vi "Display Discrete Probability Distributions.vi"() -> ()   [LabVIEW 2023]
doc: "This example VI uses Discrete PF , Discrete CDF , Discrete Inverse CDF VIs to display discrete probability (mass) functions, cumulative distribution functions, and inverse cumulative distribution functions for several discrete distributions."
uses:
  <vilib>/gmath/statdist.llb/Binomial Moments.vi
  <vilib>/gmath/statdist.llb/Binomial PF.vi
  <vilib>/gmath/statdist.llb/Binomial CDF.vi
  <vilib>/gmath/statdist.llb/Binomial Inverse CDF.vi
  <vilib>/gmath/statdist.llb/Bernoulli Moments.vi
  <vilib>/gmath/statdist.llb/Bernoulli CDF.vi
  <vilib>/gmath/statdist.llb/Bernoulli Inverse CDF.vi
  <vilib>/gmath/statdist.llb/Bernoulli PF.vi
  <vilib>/gmath/statdist.llb/Geometric Moments.vi
  <vilib>/gmath/statdist.llb/Geometric PF.vi
  <vilib>/gmath/statdist.llb/Geometric CDF.vi
  <vilib>/gmath/statdist.llb/Geometric Inverse CDF.vi
  <vilib>/gmath/statdist.llb/Hypergeometric Moments.vi
  <vilib>/gmath/statdist.llb/Hypergeometric PF.vi
  <vilib>/gmath/statdist.llb/Hypergeometric CDF.vi
  <vilib>/gmath/statdist.llb/Hypergeometric Inverse CDF.vi
  <vilib>/gmath/statdist.llb/Neg Binomial Moments.vi
  <vilib>/gmath/statdist.llb/Neg Binomial CDF.vi
  <vilib>/gmath/statdist.llb/Neg Binomial Inverse CDF.vi
  <vilib>/gmath/statdist.llb/Neg Binomial PF.vi
  <vilib>/gmath/statdist.llb/Poisson Moments.vi
  <vilib>/gmath/statdist.llb/Poisson PF.vi
  <vilib>/gmath/statdist.llb/Poisson CDF.vi
  <vilib>/gmath/statdist.llb/Poisson Inverse CDF.vi
  <vilib>/gmath/NI_Gmath.lvlib
panel:
  in  "Stop":bool
  in  "Tab Control":T1(tab)
  out "Bernoulli Inverse Cumulative Distribution Function":cluster{dbl[], i32[]}(graph)
  out "Bernoulli Cumulative Distribution Function":cluster{i32[], dbl[]}(graph)
  out "Variance (Bernoulli)":dbl
  out "Mean (Bernoulli)":dbl
  out "Bernoulli Probability Function":cluster{i32[], dbl[]}(graph)
  in  "p (Bernoulli)":dbl(slide)=0.3 min=0.0 max=1.0 scale=0.0..1.0
  out "Variance (Binomial)":dbl
  out "Mean (Binomial)":dbl
  in  "end (Binomial)":i32=20
  in  "start (Binomial)":i32
  in  "n (Binomial)":i32=13
  in  "p (Binomial)":dbl(slide)=0.3 min=0.0 max=1.0 scale=0.0..1.0
  out "Binomial Cumulative Distribution Function":cluster{i32[], dbl[]}(graph)
  out "Binomial Inverse Cumulative Distribution Function":cluster{dbl[], i32[]}(graph)
  out "Binomial Probability Function":cluster{i32[], dbl[]}(graph)
  in  "start (Geometric)":i32
  in  "end (Geometric)":i32=35
  out "Geometric Inverse Cumulative Distribution Function":cluster{dbl[], i32[]}(graph)
  out "Geometric Cumulative Distribution Function":cluster{i32[], dbl[]}(graph)
  out "Variance (Geometric)":dbl
  out "Mean (Geometric)":dbl
  out "Geometric Probability Function":cluster{i32[], dbl[]}(graph)
  in  "p (Geometric)":dbl(slide)=0.2 min=0.0 max=1.0 scale=0.0..1.0
  out "Variance (Hyper)":dbl
  out "Mean (Hyper)":dbl
  in  "n (Hyper)":i32=20
  in  "start (Hyper)":i32
  in  "end (Hyper)":i32=20
  in  "M (Hyper)":i32=31
  in  "k (Hyper)":i32=14
  out "Hypergeometric Cumulative Distribution Function":cluster{i32[], dbl[]}(graph)
  out "Hypergeometric Inverse Cumulative Distribution Function":cluster{dbl[], i32[]}(graph)
  out "Hypergeometric Probability Function":cluster{i32[], dbl[]}(graph)
  in  "start (Neg Binomial)":i32
  in  "end (Neg Binomial)":i32=40
  out "Neg Binomial Inverse Cumulative Distribution Function":cluster{dbl[], i32[]}(graph)
  in  "n (Neg Binomial)":i32=7
  out "Neg Binomial Cumulative Distribution Function":cluster{i32[], dbl[]}(graph)
  out "Variance (Neg Binomial)":dbl
  out "Mean (Neg Binomial)":dbl
  out "Neg Binomial Probability Function":cluster{i32[], dbl[]}(graph)
  in  "p (Neg Binomial)":dbl(slide)=0.4 min=0.0 max=1.0 scale=0.0..1.0
  out "Variance (Poisson)":dbl
  out "Mean (Poisson)":dbl
  in  "Lambda (Poisson)":dbl(slide)=22.0 scale=1e-08..50.0
  in  "end (Poisson)":i32=50
  in  "start (Poisson)":i32
  out "Poisson Inverse Cumulative Distribution Function":cluster{dbl[], i32[]}(graph)
  out "Poisson Cumulative Distribution Function":cluster{i32[], dbl[]}(graph)
  out "Poisson Probability Function":cluster{i32[], dbl[]}(graph)
  # "Overview: Demonstrates the use of the Discrete PF VI, Discrete CDF VI, and Discrete Inverse CDF VI.\nRequirements: LabVIEW Full Development System\nInstructions: \n1. Run the VI.\n2. Switch between tabs to explore how the parameters affect each distribution.\n3. Click Stop to stop the VI."
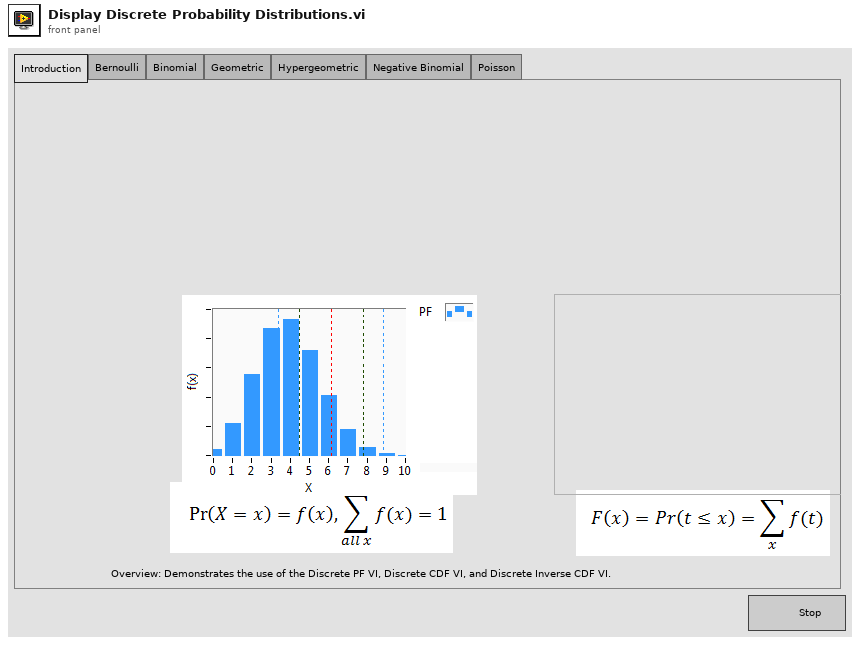
[diagram p1: front panel]
types:
  T1 = enum32{"Introduction", "Bernoulli", "Binomial", "Geometric", "Hypergeometric", "Negative Binomial", "Poisson"}
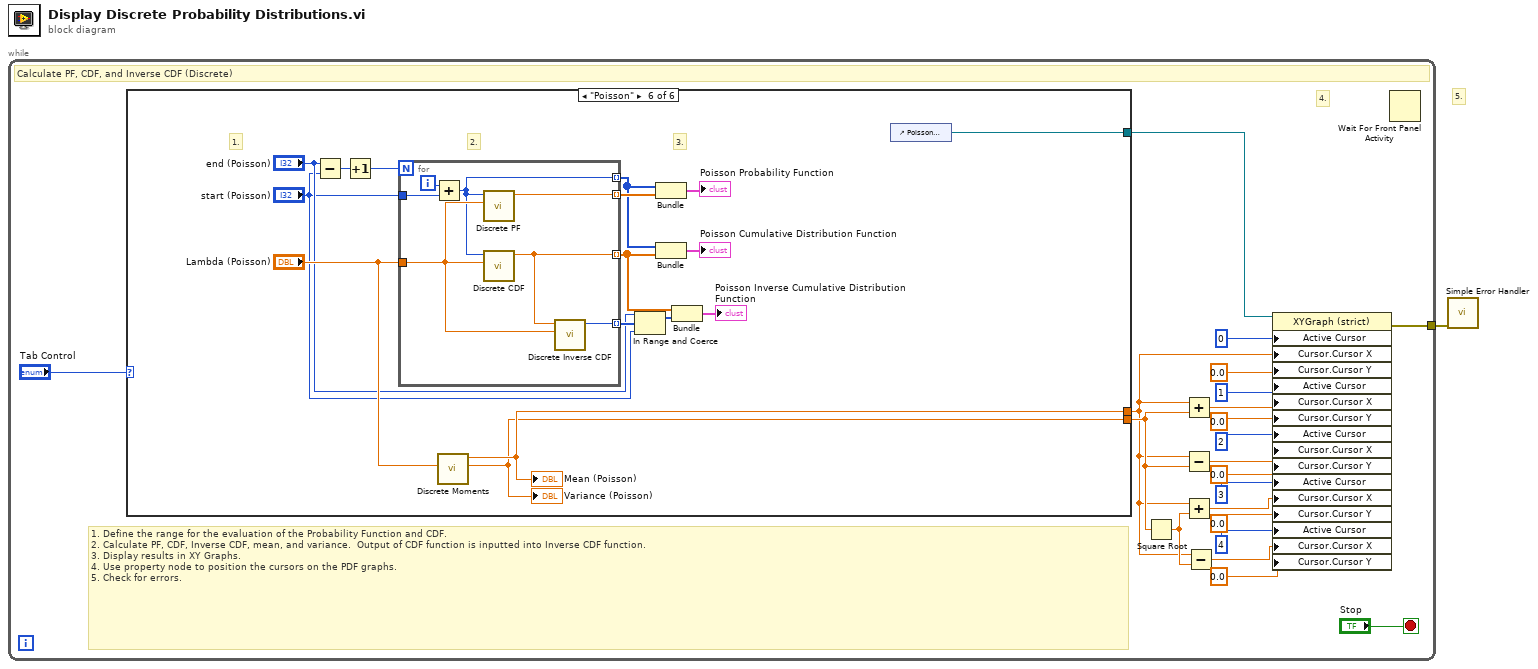
[diagram p0: block diagram]
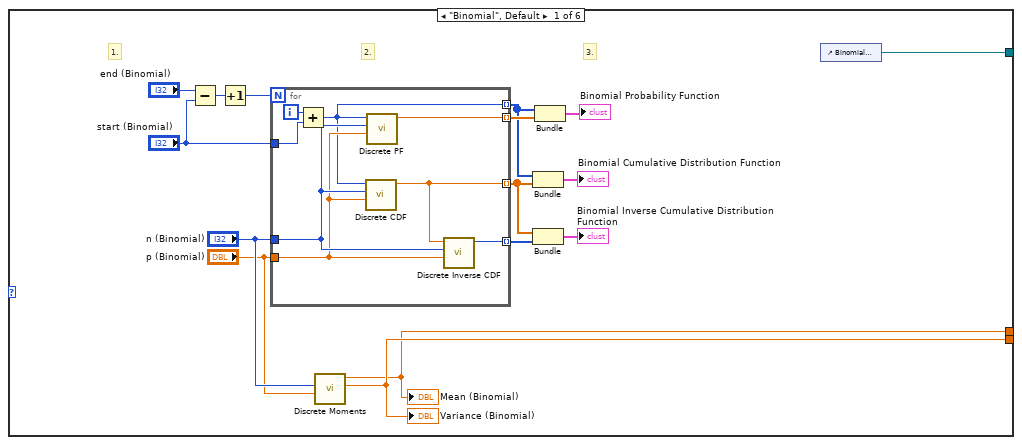
[diagram p2: hidden frame]
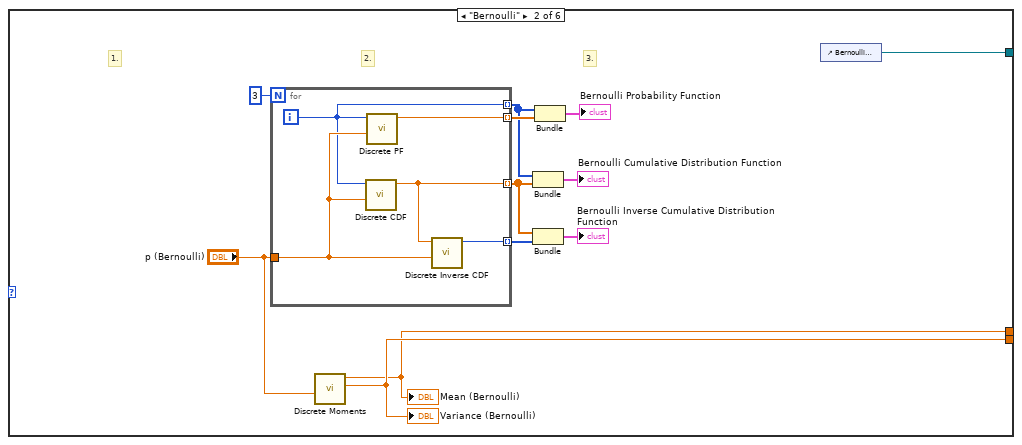
[diagram p3: hidden frame]
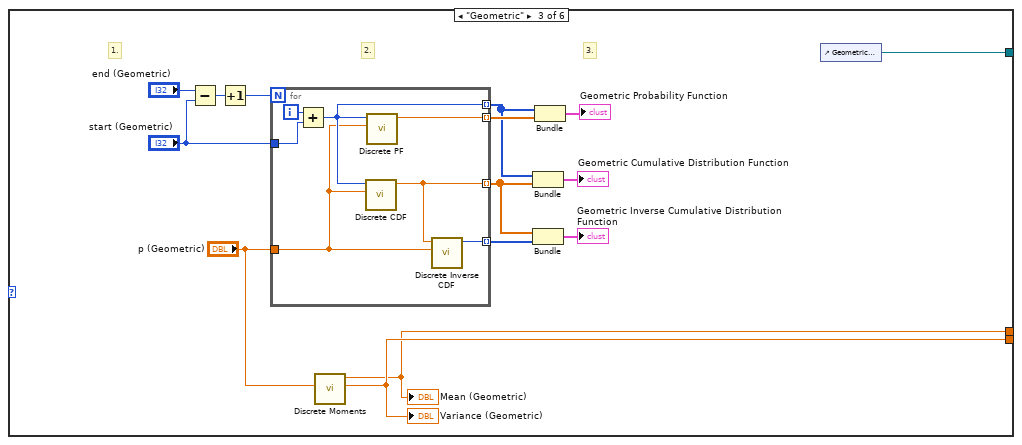
[diagram p4: hidden frame]
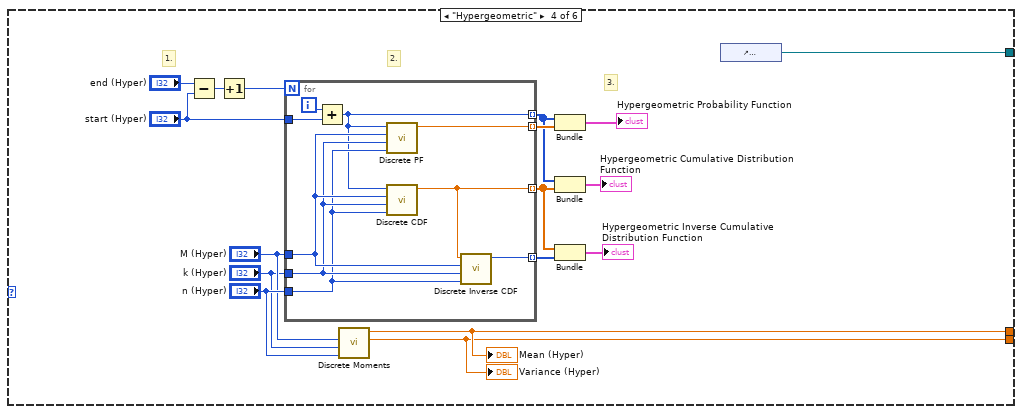
[diagram p5: hidden frame]
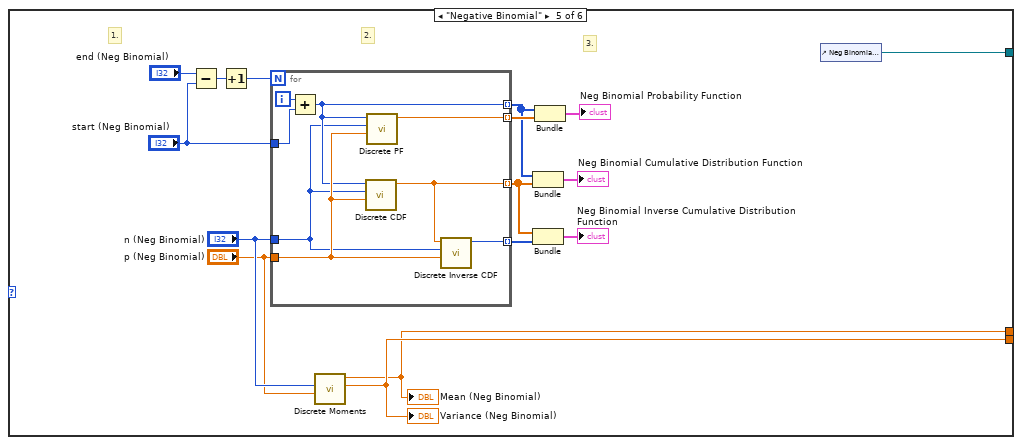
[diagram p6: hidden frame]
diagram:
  # "5."
  n1 = while {
    tunnel: [w4] -> w1
    stop <- "Stop" stop-if-true
    # "1. Define the range for the evaluation of the Probability Function and CDF.\n2. Calculate PF, CDF, Inverse CDF, mean, and variance.  Output of CDF function is inputted into Inverse CDF function.\n3. Display results in XY Graphs.\n4. Use property node to position the cursors on the PDF graphs.\n5. Check for errors."
    # "4."
    # "Calculate PF, CDF, and Inverse CDF (Discrete)"
    n2 = case shown="\"Poisson\"" "Tab Control" {
      tunnel: [w28 w49 w70 w95 w117 w144] -> w2
      tunnel: [w29 w50 w71 w94 w118 w143] -> w5
      tunnel: [w30 w51 w72 w93 w119 w145] -> w3
      frame "Binomial", Default {
        # "3."
        # "2."
        # "1."
        n3 = Subtract(x="end (Binomial)", y="start (Binomial)") -> (x-y=w24:i32)
        n4 = Increment(x=w24) -> (x+1=w23:i32)
        n5 = for {
          N: w23 -> [_]
          tunnel: [w46] -> w38 mode=indexing
          tunnel: [w44] -> w36 mode=indexing
          tunnel: [w45] -> w37 mode=indexing
          tunnel: "n (Binomial)" -> [w43]
          tunnel: "p (Binomial)" -> [w42]
          tunnel: "start (Binomial)" -> [w40]
          tunnel: [w39] -> w27 mode=indexing
          i -> [w41]
          n6 = Add(x=w41, y=w40) -> (x+y=w39:i32)
          n7 = call-poly <vilib>:"Discrete CDF.vi"("p"=w42, "n"=w43, "x"=w39) -> ("cdf(x)"=w44:dbl)  [unwired: 7 in, 1 out]
          n8 = call-poly <vilib>:"Discrete PF.vi"("p"=w42, "n"=w43, "x"=w39) -> ("prob(x)"=w46:dbl)  [unwired: 7 in, 1 out]
          n9 = call-poly <vilib>:"Discrete Inverse CDF.vi"("p"=w42, "n"=w43, "cdf(x)"=w44) -> ("x"=w45:i32)  [unwired: 7 in, 1 out]
        }
        n10 = call-poly <vilib>:"Discrete Moments.vi"("p"="p (Binomial)", "n"="n (Binomial)") -> ("variance"=w29:dbl, "mean"=w28:dbl)  [unwired: 7 in, 1 out]
        "Mean (Binomial)" <- w28
        "Variance (Binomial)" <- w29
        n11 = Bundle(w27, w36) -> (→"Binomial Cumulative Distribution Function":cluster{i32[], dbl[]})  [unwired: 1 in]
        n12 = Bundle(w36, w37) -> (→"Binomial Inverse Cumulative Distribution Function":cluster{dbl[], i32[]})  [unwired: 1 in]
        n13 = Bundle(w27, w38) -> (→"Binomial Probability Function":cluster{i32[], dbl[]})  [unwired: 1 in]
        n14 = control-ref of="Binomial Probability Function"() -> (w30:refnum<vi>)
      }
      frame "Bernoulli" {
        # "3."
        # "2."
        # "1."
        n15 = for {
          N: 3 -> [_]
          tunnel: [w63] -> w58 mode=indexing
          tunnel: [w61] -> w56 mode=indexing
          tunnel: [w62] -> w57 mode=indexing
          tunnel: "p (Bernoulli)" -> [w60]
          tunnel: [w59] -> w48 mode=indexing
          i -> [w59]
          n16 = call-poly <vilib>:"Discrete CDF.vi"("p"=w60, "x"=w59) -> ("cdf(x)"=w61:dbl)  [unwired: 8 in, 1 out]
          n17 = call-poly <vilib>:"Discrete PF.vi"("p"=w60, "x"=w59) -> ("prob(x)"=w63:dbl)  [unwired: 8 in, 1 out]
          n18 = call-poly <vilib>:"Discrete Inverse CDF.vi"("p"=w60, "cdf(x)"=w61) -> ("x"=w62:i32)  [unwired: 8 in, 1 out]
        }
        n19 = call-poly <vilib>:"Discrete Moments.vi"("p"="p (Bernoulli)") -> ("variance"=w50:dbl, "mean"=w49:dbl)  [unwired: 8 in, 1 out]
        "Mean (Bernoulli)" <- w49
        "Variance (Bernoulli)" <- w50
        n20 = Bundle(w48, w56) -> (→"Bernoulli Cumulative Distribution Function":cluster{i32[], dbl[]})  [unwired: 1 in]
        n21 = Bundle(w56, w57) -> (→"Bernoulli Inverse Cumulative Distribution Function":cluster{dbl[], i32[]})  [unwired: 1 in]
        n22 = Bundle(w48, w58) -> (→"Bernoulli Probability Function":cluster{i32[], dbl[]})  [unwired: 1 in]
        n23 = control-ref of="Bernoulli Probability Function"() -> (w51:refnum<vi>)
      }
      frame "Geometric" {
        # "3."
        # "2."
        # "1."
        n24 = Subtract(x="end (Geometric)", y="start (Geometric)") -> (x-y=w66:i32)
        n25 = Increment(x=w66) -> (x+1=w65:i32)
        n26 = for {
          N: w65 -> [_]
          tunnel: [w85] -> w78 mode=indexing
          tunnel: [w83] -> w76 mode=indexing
          tunnel: [w84] -> w77 mode=indexing
          tunnel: "p (Geometric)" -> [w79]
          tunnel: "start (Geometric)" -> [w81]
          tunnel: [w80] -> w69 mode=indexing
          i -> [w82]
          n27 = Add(x=w82, y=w81) -> (x+y=w80:i32)
          n28 = call-poly <vilib>:"Discrete CDF.vi"("p"=w79, "n"=w80) -> ("cdf(n)"=w83:dbl)  [unwired: 8 in, 1 out]
          n29 = call-poly <vilib>:"Discrete PF.vi"("p"=w79, "x"=w80) -> ("prob(x)"=w85:dbl)  [unwired: 8 in, 1 out]
          n30 = call-poly <vilib>:"Discrete Inverse CDF.vi"("p"=w79, "cdf(n)"=w83) -> ("n"=w84:i32)  [unwired: 8 in, 1 out]
        }
        n31 = call-poly <vilib>:"Discrete Moments.vi"("p"="p (Geometric)") -> ("variance"=w71:dbl, "mean"=w70:dbl)  [unwired: 8 in, 1 out]
        "Mean (Geometric)" <- w70
        "Variance (Geometric)" <- w71
        n32 = Bundle(w69, w76) -> (→"Geometric Cumulative Distribution Function":cluster{i32[], dbl[]})  [unwired: 1 in]
        n33 = Bundle(w76, w77) -> (→"Geometric Inverse Cumulative Distribution Function":cluster{dbl[], i32[]})  [unwired: 1 in]
        n34 = Bundle(w69, w78) -> (→"Geometric Probability Function":cluster{i32[], dbl[]})  [unwired: 1 in]
        n35 = control-ref of="Geometric Probability Function"() -> (w72:refnum<vi>)
      }
      frame "Hypergeometric" {
        # "3."
        # "2."
        # "1."
        n36 = Subtract(x="end (Hyper)", y="start (Hyper)") -> (x-y=w90:i32)
        n37 = Increment(x=w90) -> (x+1=w88:i32)
        n38 = for {
          N: w88 -> [_]
          tunnel: [w111] -> w102 mode=indexing
          tunnel: [w109] -> w100 mode=indexing
          tunnel: [w110] -> w101 mode=indexing
          tunnel: "M (Hyper)" -> [w108]
          tunnel: "k (Hyper)" -> [w107]
          tunnel: "n (Hyper)" -> [w106]
          tunnel: "start (Hyper)" -> [w104]
          tunnel: [w103] -> w86 mode=indexing
          i -> [w105]
          n39 = Add(x=w105, y=w104) -> (x+y=w103:i32)
          n40 = call-poly <vilib>:"Discrete PF.vi"("n"=w106, "k"=w107, "M"=w108, "x"=w103) -> ("prob(x)"=w111:dbl)  [unwired: 6 in, 1 out]
          n41 = call-poly <vilib>:"Discrete CDF.vi"("n"=w106, "k"=w107, "M"=w108, "x"=w103) -> ("cdf(x)"=w109:dbl)  [unwired: 6 in, 1 out]
          n42 = call-poly <vilib>:"Discrete Inverse CDF.vi"("n"=w106, "k"=w107, "M"=w108, "cdf(x)"=w109) -> ("x"=w110:i32)  [unwired: 6 in, 1 out]
        }
        n43 = call-poly <vilib>:"Discrete Moments.vi"("n"="n (Hyper)", "k"="k (Hyper)", "M"="M (Hyper)") -> ("variance"=w94:dbl, "mean"=w95:dbl)  [unwired: 6 in, 1 out]
        "Mean (Hyper)" <- w95
        "Variance (Hyper)" <- w94
        n44 = Bundle(w86, w102) -> (→"Hypergeometric Probability Function":cluster{i32[], dbl[]})  [unwired: 1 in]
        n45 = Bundle(w86, w100) -> (→"Hypergeometric Cumulative Distribution Function":cluster{i32[], dbl[]})  [unwired: 1 in]
        n46 = Bundle(w100, w101) -> (→"Hypergeometric Inverse Cumulative Distribution Function":cluster{dbl[], i32[]})  [unwired: 1 in]
        n47 = control-ref of="Hypergeometric Probability Function"() -> (w93:refnum<vi>)
      }
      frame "Negative Binomial" {
        # "3."
        # "2."
        # "1."
        n48 = Subtract(x="end (Neg Binomial)", y="start (Neg Binomial)") -> (x-y=w113:i32)
        n49 = Increment(x=w113) -> (x+1=w112:i32)
        n50 = for {
          N: w112 -> [_]
          tunnel: [w135] -> w127 mode=indexing
          tunnel: [w133] -> w125 mode=indexing
          tunnel: [w134] -> w126 mode=indexing
          tunnel: "n (Neg Binomial)" -> [w128]
          tunnel: "p (Neg Binomial)" -> [w132]
          tunnel: "start (Neg Binomial)" -> [w130]
          tunnel: [w129] -> w116 mode=indexing
          i -> [w131]
          n51 = Add(x=w131, y=w130) -> (x+y=w129:i32)
          n52 = call-poly <vilib>:"Discrete CDF.vi"("p"=w132, "x"=w128, "y"=w129) -> ("cdf(y)"=w133:dbl)  [unwired: 7 in, 1 out]
          n53 = call-poly <vilib>:"Discrete PF.vi"("p"=w132, "x"=w128, "y"=w129) -> ("prob(y)"=w135:dbl)  [unwired: 7 in, 1 out]
          n54 = call-poly <vilib>:"Discrete Inverse CDF.vi"("p"=w132, "x"=w128, "cdf(y)"=w133) -> ("y"=w134:i32)  [unwired: 7 in, 1 out]
        }
        n55 = call-poly <vilib>:"Discrete Moments.vi"("p"="p (Neg Binomial)", "x"="n (Neg Binomial)") -> ("variance"=w118:dbl, "mean"=w117:dbl)  [unwired: 7 in, 1 out]
        "Mean (Neg Binomial)" <- w117
        "Variance (Neg Binomial)" <- w118
        n56 = Bundle(w116, w125) -> (→"Neg Binomial Cumulative Distribution Function":cluster{i32[], dbl[]})  [unwired: 1 in]
        n57 = Bundle(w125, w126) -> (→"Neg Binomial Inverse Cumulative Distribution Function":cluster{dbl[], i32[]})  [unwired: 1 in]
        n58 = Bundle(w116, w127) -> (→"Neg Binomial Probability Function":cluster{i32[], dbl[]})  [unwired: 1 in]
        n59 = control-ref of="Neg Binomial Probability Function"() -> (w119:refnum<vi>)
      }
      frame "Poisson" {
        # "3."
        # "2."
        # "1."
        n60 = Subtract(x="end (Poisson)", y="start (Poisson)") -> (x-y=w142:i32)
        n61 = Increment(x=w142) -> (x+1=w141:i32)
        n62 = for {
          N: w141 -> [_]
          tunnel: [w158] -> w151 mode=indexing
          tunnel: [w156] -> w150 mode=indexing
          tunnel: [w157] -> w139 mode=indexing
          tunnel: "Lambda (Poisson)" -> [w155]
          tunnel: "start (Poisson)" -> [w153]
          tunnel: [w152] -> w140 mode=indexing
          i -> [w154]
          n63 = Add(x=w154, y=w153) -> (x+y=w152:i32)
          n64 = call-poly <vilib>:"Discrete PF.vi"("lambda"=w155, "x"=w152) -> ("prob(x)"=w158:dbl)  [unwired: 8 in, 1 out]
          n65 = call-poly <vilib>:"Discrete CDF.vi"("lambda"=w155, "x"=w152) -> ("cdf(x)"=w156:dbl)  [unwired: 8 in, 1 out]
          n66 = call-poly <vilib>:"Discrete Inverse CDF.vi"("lambda"=w155, "cdf(x)"=w156) -> ("x"=w157:i32)  [unwired: 8 in, 1 out]
        }
        n67 = call-poly <vilib>:"Discrete Moments.vi"("lambda"="Lambda (Poisson)") -> ("variance"=w143:dbl, "mean"=w144:dbl)  [unwired: 8 in, 1 out]
        "Mean (Poisson)" <- w144
        "Variance (Poisson)" <- w143
        n68 = In Range and Coerce(upper limit="end (Poisson)", x=w139, lower limit="start (Poisson)") -> (coerced(x)=w138:i32[])  [unwired: 1 out]
        n69 = Bundle(w140, w151) -> (→"Poisson Probability Function":cluster{i32[], dbl[]})  [unwired: 1 in]
        n70 = Bundle(w140, w150) -> (→"Poisson Cumulative Distribution Function":cluster{i32[], dbl[]})  [unwired: 1 in]
        n71 = Bundle(w150, w138) -> (→"Poisson Inverse Cumulative Distribution Function":cluster{dbl[], i32[]})  [unwired: 1 in]
        n72 = control-ref of="Poisson Probability Function"() -> (w145:refnum<vi>)
      }
    }
    n73 = Square Root(x=w5) -> (sqrt(x)=w8:dbl)
    n74 = Add(x=w2, y=w5) -> (x+y=w11:dbl)
    n75 = Subtract(x=w2, y=w5) -> (x-y=w10:dbl)
    n76 = Add(x=w2, y=w8) -> (x+y=w9:dbl)
    n77 = Subtract(x=w2, y=w8) -> (x-y=w7:dbl)
    n78 = property on="Property Node" class="XYGraph (strict)"(reference=w3, "Active Cursor"=u32 0, "Cursor.Cursor X"=w2, "Cursor.Cursor Y"=0.0 ("Cursor.Cursor Position:Cursor Y"), "Active Cursor"=u32 1, "Cursor.Cursor X"=w11, "Cursor.Cursor Y"=0.0 ("Cursor.Cursor Position:Cursor Y"), "Active Cursor"=u32 2, "Cursor.Cursor X"=w10, "Cursor.Cursor Y"=0.0 ("Cursor.Cursor Position:Cursor Y"), "Active Cursor"=u32 3, "Cursor.Cursor X"=w9, "Cursor.Cursor Y"=0.0 ("Cursor.Cursor Position:Cursor Y"), "Active Cursor"=u32 4, "Cursor.Cursor X"=w7, "Cursor.Cursor Y"=0.0 ("Cursor.Cursor Position:Cursor Y")) -> (error out=w4:errorcluster)  [unwired: 1 in, 1 out]
    n79 = Wait For Front Panel Activity() -> ()  [unwired: 3 in, 1 out]
  }
  n80 = call <vilib>:"Simple Error Handler.vi"("error in (no error)"=w1) -> ()  [unwired: 4 in, 5 out]
